vi "FPGA-Sample_currents_read_fractional_pulses.vi"() -> ()   [LabVIEW 2013]
uses:
  <vilib>/Platform/TimedLoop/XDataNode/timing_clust.ctl
  <vilib>/Platform/TimedLoop/XDataNode/nitl_modes.ctl
  <vilib>/Platform/TimedLoop/XDataNode/wakeup.ctl
  <vilib>/rvi/FXPMathLib/basic elements/FxpIntAccumulator/subVIs/nifxpmath_IntAccumulator_SimConfig.ctl
  <vilib>/rvi/Emulation/niFpgaSctlEmulationGetInTimedLoop.vi
  <vilib>/rvi/Emulation/niFpgaEmulationReportErrorSimple.vi
  <vilib>/rvi/Emulation/niFpgaGetClockAttributes.vi
  <vilib>/rvi/Emulation/niFpgaCriticalErrorInLSC.vi
  <vilib>/rvi/eio/common/nirviEmuTemplateMethod_errors.vi
  <vilib>/rvi/Emulation/niFpgaProcessEmulError.vi
  <vilib>/rvi/FXPMathLib/basic elements/FxpIntAccumulator/simVIs/DllFxpIntAccumulator_sub.vi
  <vilib>/Platform/TimedLoop/XDataNode/XDataNode.xnode
  <vilib>/eio/EIONode/EIONode.xnode
  <vilib>/rvi/FXPMathLib/basic elements/FxpIntAccumulator/XNode/nifxpmath_IntAccumulator.xnode
  <vilib>/Platform/TimedLoop/XDataNode/XDNodeRunTimeDep.lvlib
panel:
  out "mA*seconds (input 1)":fxp<+/-,64,28>
  out "mA*seconds (input 2)":fxp<+/-,64,28>
  out "Sampling in progress 2":bool
  out "Sampling in progress 1":bool
  out "Gate time 2":u64
  out "whole pulse time 2":u64
  out "Whole pulses 2":u64
  in  "Sample period Input 1":u64=200000000
  out "Whole pulses 1":u64
  out "whole pulse time 1":u64
  out "Gate time 1":u64
  in  "Sample period Input 0":u64=200000000
  in  "Begin pulse sampling":bool
  out "Currents":fxp<+/-,24,-4>[](array[numeric])
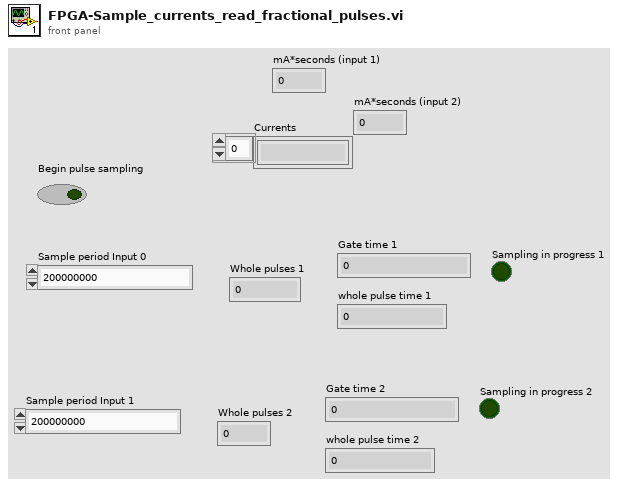
[diagram p1: front panel]
types:
  T1 = typedef "XDNodeRunTimeDep.lvlib/timing_clust.ctl" = cluster{"Expected End [f-1]":u64, "Actual End [f-1]":u64, "Finished Late? [f-1]":bool, "Expected End [i-1]":u64, "Actual End [i-1]":u64, "Finished Late? [i-1]":bool, "Expected Start [i]":u64, "Actual Start [i]":u64, "Expected Start [f]":u64, "Actual Start [f]":u64, "Source Name":string, "Structure Name":string, "Period":i64, "Deadline":i64, "Offset":i64, "Start":i64, "Priority":i32, "Timeout":i32, "Mode":T2, "Wakeup Reason":T3, "Error":errorcluster, "Source Type":string, "Secondary Source Type":string, "Global End Time":u64, "Global Start Time":u64, "Frame Duration":u64, "Iteration Duration":u64, "Assigned CPU":i32, "I/O Scan Engine Mode":u32}
  T2 = typedef "XDNodeRunTimeDep.lvlib/nitl_modes.ctl" = enum32{"No Change", "Process missed periods, maintain original phase", "Discard missed periods, maintain original phase", "Process missed periods, ignore original phase", "Discard missed periods, ignore original phase"}
  T3 = typedef "XDNodeRunTimeDep.lvlib/wakeup.ctl" = enum32{"Normal", "Aborted", "Asynchronous wakeup", "Timing source error", "Timed loop error", "Timeout"}
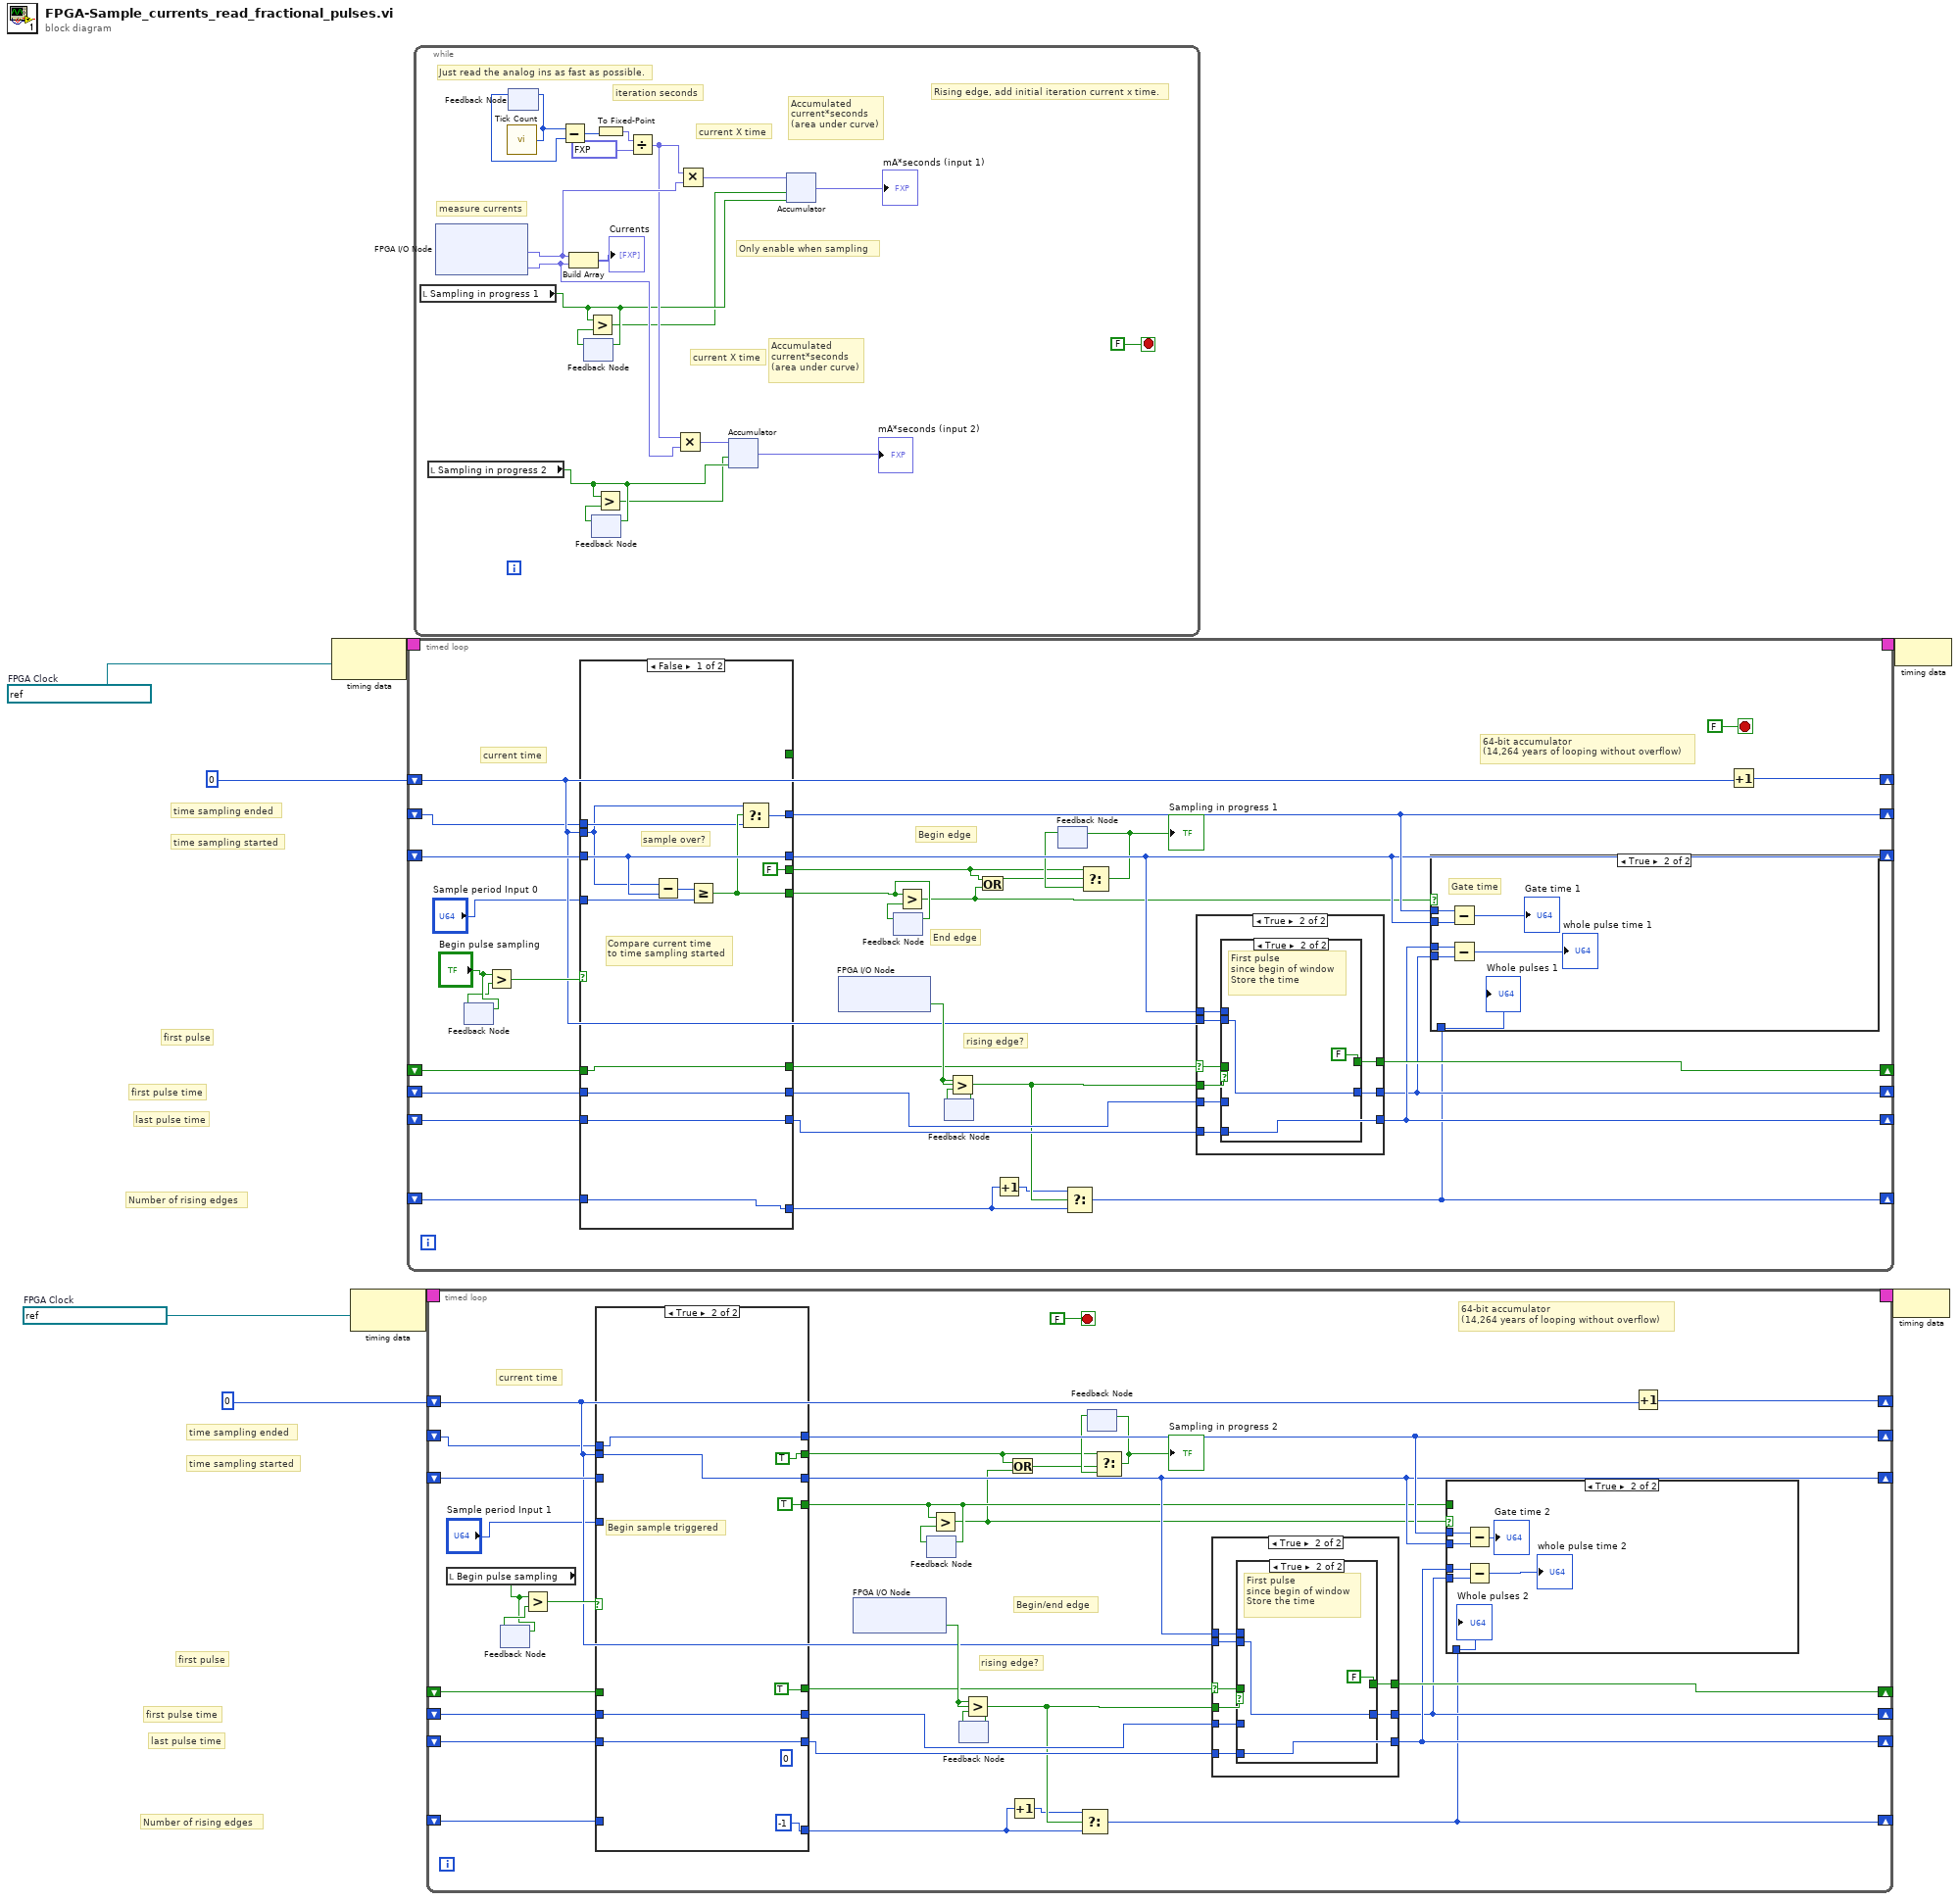
[diagram p0: block diagram]
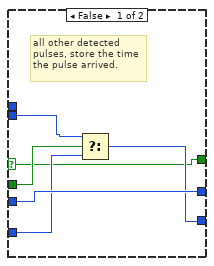
[diagram p3: hidden frame]
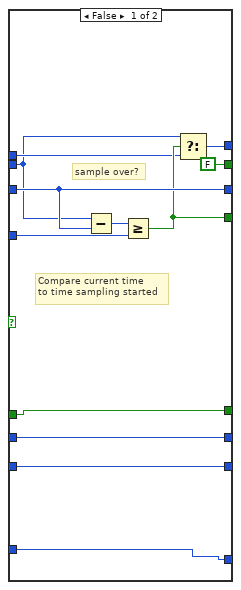
[diagram p5: hidden frame]
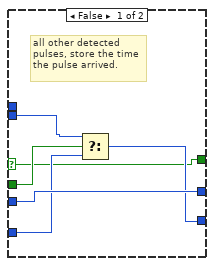
[diagram p7: hidden frame]
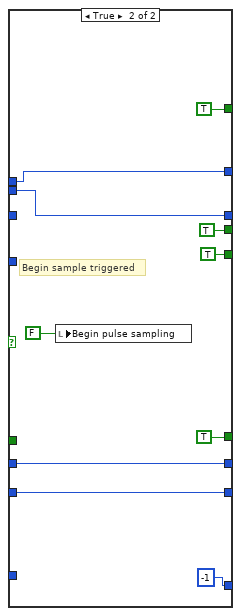
[diagram p9: hidden frame]
diagram:
  w1 = refnum<k21> "40 MHz Onboard Clock"  # FPGA Clock
  w6 = refnum<k21> "40 MHz Onboard Clock"  # FPGA Clock
  # "time sampling ended"
  # "time sampling started"
  # "Number of rising edges"
  # "last pulse time"
  # "first pulse time"
  # "first pulse"
  # "time sampling ended"
  # "time sampling started"
  # "Number of rising edges"
  # "last pulse time"
  # "first pulse time"
  # "first pulse"
  n1 = node-c288(w6) -> (w8:T1)
  n2 = node-c288(w1) -> (w4:T1)
  n3 = timed-loop {
    timing: w8 -> [_]
    timing-out: [_] -> w7
    shift-right: [w24] -> _
    shift-left: _ -> [w38]
    shift-right: [w35] -> _
    shift-left: u64 0 -> [w34]
    shift-right: [w22] -> _
    shift-left: _ -> [w31]
    shift-right: [w27] -> _
    shift-left: _ -> [w33]
    shift-right: [w23] -> _
    shift-left: _ -> [w29]
    shift-right: [w25] -> _
    shift-left: _ -> [w26]
    shift-right: [w17] -> _
    shift-left: _ -> [w20]
    stop <- FALSE stop-if-true
    # "Begin edge"
    # "End edge"
    # "current time"
    # "64-bit accumulator\n(14,264 years of looping without overflow)"
    # "rising edge?"
    n4 = feedback-in #1("Begin pulse sampling") -> ()
    n5 = feedback #1() -> (w40:bool)  [unwired: 1 in]
    n6 = Greater?(x="Begin pulse sampling", y=w40) -> (0:w39:bool)
    n7 = case shown="False" w39 {
      tunnel: w34 -> [w70 w88]
      tunnel: [w79 w88] -> w24
      tunnel: w38 -> [w79 _]
      tunnel: "Sample period Input 0" -> [w77 _]
      tunnel: [w73 TRUE] -> w14
      tunnel: w33 -> [w76 _]
      tunnel: [w76 TRUE ("x > y?")] -> w32
      tunnel: w31 -> [w75 w86]
      tunnel: [w75 w86] -> w30
      tunnel: w29 -> [w74 w85]
      tunnel: [w74 w85] -> w28
      tunnel: [w72 w84] -> w25
      tunnel: w26 -> [w71 w84]
      tunnel: [w69 i64 -1] -> w19
      tunnel: w20 -> [w69 _]
      tunnel: [FALSE TRUE] -> w11
      tunnel: [_ TRUE ("load (F)")] -> _
      frame False {
        # "sample over?"
        # "Compare current time\nto time sampling started"
        n8 = Subtract(x=w70, y=w79) -> (x-y=w78:u64)
        n9 = Greater Or Equal?(x=w78, y=w77) -> (x >= y?=w73:bool)
        n10 = Select(t=w70, s=w73, f=w71) -> (s? t:f=w72:u64)
      }
      frame True {
        # "Begin sample triggered"
        n11 = local write "Begin pulse sampling"(FALSE ("Begin pulse sampling")) -> ()
      }
    }
    n12 = xnode "FPGA I/O Node"() -> ("Mod1/DI0"=w37:bool)  [unwired: 1 in, 1 out]
    n13 = feedback #2() -> (w16:bool)  [unwired: 1 in]
    n14 = feedback-in #2(w14) -> ()
    n15 = Greater?(x=w14, y=w16) -> (0:w10:bool)
    n16 = feedback-in #3(w37) -> ()
    n17 = feedback #3() -> (w36:bool)  [unwired: 1 in]
    n18 = Greater?(x=w37, y=w36) -> (0:w21:bool)
    n19 = Or(x=w11, y=w10) -> (x .or. y?=w9:bool)
    n20 = Increment(x=w19) -> (x+1=w18:i64)
    n21 = feedback #4() -> (w12:bool)  [unwired: 1 in]
    n22 = Select(t=w18, s=w21, f=w19) -> (s? t:f=w17:i64)
    n23 = Select(t=w11, s=w9, f=w12) -> (s? t:f=w13:bool)
    "Sampling in progress 1" <- w13
    n24 = feedback-in #4(w13) -> ()
    n25 = case shown="True" w32 {
      selector: w32 -> [w50 w57]
      tunnel: w21 -> [w53 w59]
      tunnel: w34 -> [w54 w63]
      tunnel: [w55 w61] -> w22
      tunnel: w30 -> [w55 w62]
      tunnel: w28 -> [w52 w60]
      tunnel: [w51 w60] -> w23
      tunnel: w24 -> [_ w58]
      tunnel: [w50 w56] -> w27
      frame False {
        # "all other detected\npulses, store the time\nthe pulse arrived."
        n26 = Select(t=w54, s=w53, f=w52) -> (s? t:f=w51:u64)
      }
      frame True {
        n27 = case shown="True" w59 {
          tunnel: w63 -> [_ w67]
          tunnel: w62 -> [w65 _]
          tunnel: [w65 w67] -> w61
          tunnel: w60 -> [_ _]
          tunnel: w58 -> [_ _]
          tunnel: w57 -> [w64 _]
          tunnel: [w64 FALSE] -> w56
          frame False {
          }
          frame True {
            # "First pulse\nsince begin of window\nStore the time"
          }
        }
      }
    }
    n28 = case shown="True" w10 {
      tunnel: w25 -> [_ w49]
      tunnel: w24 -> [_ w48]
      tunnel: w23 -> [_ w46]
      tunnel: w22 -> [_ w45]
      tunnel: w17 -> [_ w43]
      frame False {
      }
      frame True {
        # "Gate time"
        n29 = Subtract(x=w49, y=w48) -> (x-y=→"Gate time 1":u64)
        n30 = Subtract(x=w46, y=w45) -> (x-y=→"whole pulse time 1":u64)
        "Whole pulses 1" <- w43
      }
    }
    n31 = Increment(x=w34) -> (x+1=w35:u64)
  }
  n32 = while {
    stop <- FALSE stop-if-true
    # "Accumulated\ncurrent*seconds \n(area under curve)"
    # "current X time"
    # "Rising edge, add initial iteration current x time."
    # "Only enable when sampling"
    # "Accumulated\ncurrent*seconds \n(area under curve)"
    # "current X time"
    # "iteration seconds"
    # "Just read the analog ins as fast as possible."
    # "measure currents"
    n33 = local read "Sampling in progress 1"() -> (w99:bool)
    n34 = local read "Sampling in progress 2"() -> (w96:bool)
    n35 = xnode "FPGA I/O Node"() -> ("Mod2/AI0"=w106:fxp<+/-,24,-4>, "Mod2/AI1"=w101:fxp<+/-,24,-4>)  [unwired: 2 in, 2 out]
    n36 = call "Tick Count"() -> ("Tick Count(uSec)"=w109:u32)
    n37 = feedback-in #5(w109) -> ()
    n38 = feedback #5() -> (w108:u32)  [unwired: 1 in]
    n39 = Subtract(x=w109, y=w108) -> (x-y=w105:u32)
    n40 = Build Array(w106, w101) -> (→"Currents":fxp<+/-,24,-4>[])
    n41 = feedback #6() -> (w107:bool)  [unwired: 1 in]
    n42 = feedback-in #6(w99) -> ()
    n43 = Greater?(x=w99, y=w107) -> (0:w98:bool)
    n44 = feedback #7() -> (w102:bool)  [unwired: 1 in]
    n45 = feedback-in #7(w96) -> ()
    n46 = Greater?(x=w96, y=w102) -> (0:w94:bool)
    n47 = To Fixed-Point(number=w105) -> (fixed-point=w104:fxp<+,32,32>)  [unwired: 1 in]
    n48 = Divide(x=w104, y=fxp<+,32,32> 1000000.0) -> (x/y=w100:fxp<+,64,32>)
    n49 = Multiply(x=w100, y=w101) -> (x*y=w95:fxp<+/-,64,28>)
    n50 = Multiply(x=w100, y=w106) -> (x*y=w97:fxp<+/-,64,28>)
    n51 = xnode "Accumulator"("x"=w95, "load (F)"=w94, "enable (T)"=w96) -> ("s"=→"mA*seconds (input 2)":fxp<+/-,64,28>)  [unwired: 2 in, 1 out]
    n52 = xnode "Accumulator"("x"=w97, "load (F)"=w98, "enable (T)"=w99) -> ("s"=→"mA*seconds (input 1)":fxp<+/-,64,28>)  [unwired: 2 in, 1 out]
  }
  n53 = timed-loop {
    timing: w4 -> [_]
    timing-out: [_] -> w3
    shift-right: [w182] -> _
    shift-left: _ -> [w196]
    shift-right: [w193] -> _
    shift-left: u64 0 -> [w192]
    shift-right: [w180] -> _
    shift-left: _ -> [w189]
    shift-right: [w185] -> _
    shift-left: _ -> [w191]
    shift-right: [w181] -> _
    shift-left: _ -> [w187]
    shift-right: [w183] -> _
    shift-left: _ -> [w184]
    shift-right: [w175] -> _
    shift-left: _ -> [w178]
    stop <- FALSE stop-if-true
    # "Begin/end edge"
    # "current time"
    # "64-bit accumulator\n(14,264 years of looping without overflow)"
    # "rising edge?"
    n54 = local read "Begin pulse sampling"() -> (w173:bool)
    n55 = feedback-in #8(w173) -> ()
    n56 = feedback #8() -> (w198:bool)  [unwired: 1 in]
    n57 = Greater?(x=w173, y=w198) -> (0:w197:bool)
    n58 = case shown="True" w197 {
      tunnel: w192 -> [w227 w244]
      tunnel: [w236 w244] -> w182
      tunnel: w196 -> [w236 _]
      tunnel: "Sample period Input 1" -> [w234 _]
      tunnel: [w230 TRUE] -> w171
      tunnel: w191 -> [w233 _]
      tunnel: [w233 TRUE ("x > y?")] -> w190
      tunnel: w189 -> [w232 w242]
      tunnel: [w232 w242] -> w188
      tunnel: w187 -> [w231 w241]
      tunnel: [w231 w241] -> w186
      tunnel: [w229 w240] -> w183
      tunnel: w184 -> [w228 w240]
      tunnel: [w226 i64 -1] -> w177
      tunnel: w178 -> [w226 _]
      tunnel: [FALSE TRUE] -> w167
      frame False {
        # "sample over?"
        # "Compare current time\nto time sampling started"
        n59 = Subtract(x=w227, y=w236) -> (x-y=w235:u64)
        n60 = Greater Or Equal?(x=w235, y=w234) -> (x >= y?=w230:bool)
        n61 = Select(t=w227, s=w230, f=w228) -> (s? t:f=w229:u64)
      }
      frame True {
        (unwired) u64 0
        # "Begin sample triggered"
      }
    }
    n62 = xnode "FPGA I/O Node"() -> ("Mod1/DI1"=w195:bool)  [unwired: 1 in, 1 out]
    n63 = feedback #9() -> (w174:bool)  [unwired: 1 in]
    n64 = feedback-in #9(w171) -> ()
    n65 = Greater?(x=w171, y=w174) -> (0:w168:bool)
    n66 = feedback-in #10(w195) -> ()
    n67 = feedback #10() -> (w194:bool)  [unwired: 1 in]
    n68 = Greater?(x=w195, y=w194) -> (0:w179:bool)
    n69 = Or(x=w167, y=w168) -> (x .or. y?=w166:bool)
    n70 = Increment(x=w177) -> (x+1=w176:i64)
    n71 = Select(t=w176, s=w179, f=w177) -> (s? t:f=w175:i64)
    n72 = feedback #11() -> (w170:bool)  [unwired: 1 in]
    n73 = Select(t=w167, s=w166, f=w170) -> (s? t:f=w169:bool)
    "Sampling in progress 2" <- w169
    n74 = feedback-in #11(w169) -> ()
    n75 = case shown="True" w190 {
      selector: w190 -> [w207 w214]
      tunnel: w179 -> [w210 w216]
      tunnel: w192 -> [w211 w220]
      tunnel: [w212 w218] -> w180
      tunnel: w188 -> [w212 w219]
      tunnel: w186 -> [w209 w217]
      tunnel: [w208 w217] -> w181
      tunnel: w182 -> [_ w215]
      tunnel: [w207 w213] -> w185
      frame False {
        # "all other detected\npulses, store the time\nthe pulse arrived."
        n76 = Select(t=w211, s=w210, f=w209) -> (s? t:f=w208:u64)
      }
      frame True {
        n77 = case shown="True" w216 {
          tunnel: w220 -> [_ w224]
          tunnel: w219 -> [w222 _]
          tunnel: [w222 w224] -> w218
          tunnel: w217 -> [_ _]
          tunnel: w215 -> [_ _]
          tunnel: w214 -> [w221 _]
          tunnel: [w221 FALSE] -> w213
          frame False {
          }
          frame True {
            # "First pulse\nsince begin of window\nStore the time"
          }
        }
      }
    }
    n78 = case shown="True" w168 {
      tunnel: w183 -> [_ w206]
      tunnel: w182 -> [_ w205]
      tunnel: w181 -> [_ w203]
      tunnel: w180 -> [_ w202]
      tunnel: w175 -> [_ w200]
      tunnel: w171 -> [_ _]
      frame False {
      }
      frame True {
        n79 = Subtract(x=w206, y=w205) -> (x-y=→"Gate time 2":u64)
        n80 = Subtract(x=w203, y=w202) -> (x-y=→"whole pulse time 2":u64)
        "Whole pulses 2" <- w200
      }
    }
    n81 = Increment(x=w192) -> (x+1=w193:u64)
  }
  n82 = node-c288(w3) -> ()
  n83 = node-c288(w7) -> ()
